vi "fgv_imgbuff_4stream.vi"(7 "cmd":enum16{"cread", "read", "close"}(ring), 8 "error in (no error)":errorcluster caption="error in") -> (0 "error out":errorcluster, 3 "img out":T1[](array[typedef]))   [LabVIEW 2019]
uses:
  <vilib>/vision/Image Controls.llb/IMAQ Image.ctl
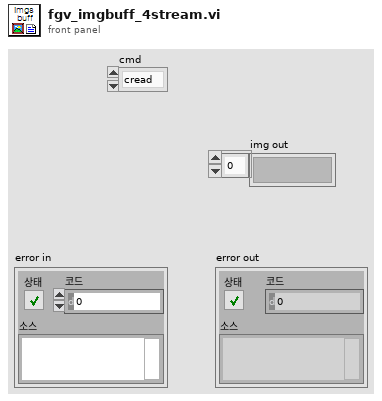
[diagram p1: front panel]
types:
  T1 = typedef "IMAQ Image.ctl" = refnum<image>
  T2 = typedef "Image Type" = u32
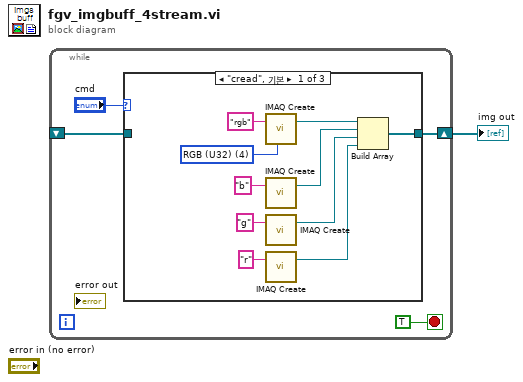
[diagram p0: block diagram]
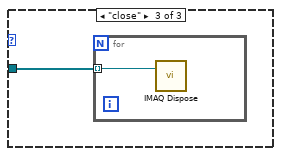
[diagram p3: hidden frame]
diagram:
  n1 = while {
    shift-right: [w3] -> w1
    shift-left: _ -> [w2]
    stop <- TRUE stop-if-true
    n2 = case shown="\"cread\", 기본" "cmd" {
      tunnel: [w6 w16 _] -> w3
      tunnel: w2 -> [_ w16 w17]
      frame "cread", Default {
        w11 = T2 4 items=["Grayscale (U8)", "Grayscale (I16)", "Grayscale (SGL)", "Complex (CSG)", "RGB (U32)", "HSL (U32)", "RGB (U64)", "Grayscale (U16)"] ("Image Type")
        n3 = call "IMAQ Create"("Image Name"="rgb", "Image Type"=w11) -> ("New Image"=w7:T1)  [unwired: 3 in, 1 out]
        n4 = call "IMAQ Create"("Image Name"="b") -> ("New Image"=w8:T1)  [unwired: 4 in, 1 out]
        n5 = call "IMAQ Create"("Image Name"="g") -> ("New Image"=w9:T1)  [unwired: 4 in, 1 out]
        n6 = call "IMAQ Create"("Image Name"="r") -> ("New Image"=w10:T1)  [unwired: 4 in, 1 out]
        n7 = Build Array(w7, w8, w9, w10) -> (w6:T1[])
      }
      frame "read" {
      }
      frame "close" {
        n8 = for {
          tunnel: w17 -> [w18] mode=indexing
          n9 = call "IMAQ Dispose"("Image"=w18) -> ()  [unwired: 5 in, 1 out]
        }
      }
    }
  }
  "img out" <- w1
